vi "AO SCTR with Digital Out Engine.vi"(0 "Unique Notifier Name":string, 11 "AO PFI Lines":string[](array[string])) -> ()   [LabVIEW 2016]
uses:
  AO SCTR Type Defs/AO SCTR Notifier Type.ctl
  AO SCTR Type Defs/AO SCTR Actions.ctl
  <vilib>/DAQmx/write.llb/DAQmx Write (Analog DBL 1Chan 1Samp).vi
  <vilib>/Analysis/1siggen.llb/Ramp Pattern by Samples.vi
  <vilib>/DAQmx/write.llb/DAQmx Write (Analog 1D DBL 1Chan NSamp).vi
  <vilib>/DAQmx/create/channels.llb/DAQmx Create Channel (CO-Pulse Generation-Time).vi
  <vilib>/DAQmx/create/channels.llb/DAQmx Create Channel (AO-Voltage-Basic).vi
  <vilib>/DAQmx/miscellaneous.llb/DAQmx Fill In Error Info.vi
  <vilib>/DAQmx/configure/timing.llb/DAQmx Timing (Sample Clock).vi
  <resource>/objmgr/daqmx.rc
  <vilib>/Analysis/NI_AALBase.lvlib
panel:
  in  "Initial Delay":dbl format="%.6f"
  in  "Exposure Time (s)":dbl
  in  "Disable Input":bool
  out "Running":bool
  in  "Load":bool
  in  "Save":bool
  in  "Quit":bool
  in  "Waveform Settings":T1={"Actions"=enum."Stop at Offset", "Offset (V)"=-0.61, "Amplititude (V)"=0.524, "Samples Per Channel"=2280, "Start Delay (ms)"=20.0, "Running?"=FALSE} {"Amplititude (V)" format="%#_13g"; "Offset (V)" format="%#_13g"; "Start Delay (ms)" format="%#_13g"}
  out "Waveform Graph":dbl[](graph)
  out "Actual Sample Rate":dbl=10000.0 format="%0.2f"
  # "AO Line. Example: Dev1/ao1\nPFI (Trigger) Line. Example: /Dev1/PFI0\nCounter. Example: Dev1/ctr0"
  # "For debugging only."
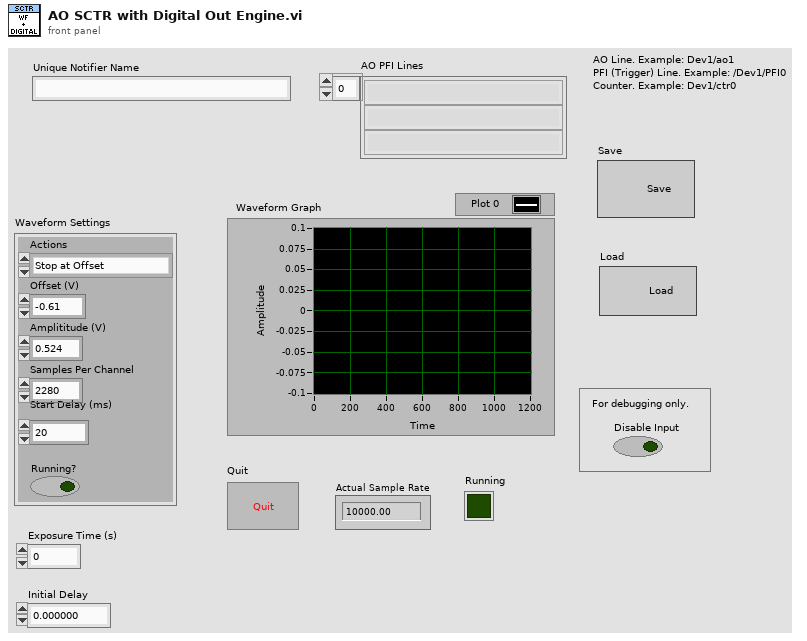
[diagram p1: front panel]
types:
  T1 = typedef "AO SCTR Notifier Type.ctl" = cluster{"Actions":T2, "Offset (V)":dbl, "Amplititude (V)":dbl, "Samples Per Channel":i32, "Start Delay (ms)":dbl, "Running?":bool}
  T2 = typedef "AO SCTR Actions.ctl" = enum16{"Stop at Offset", "Update and Run", "Quit"}
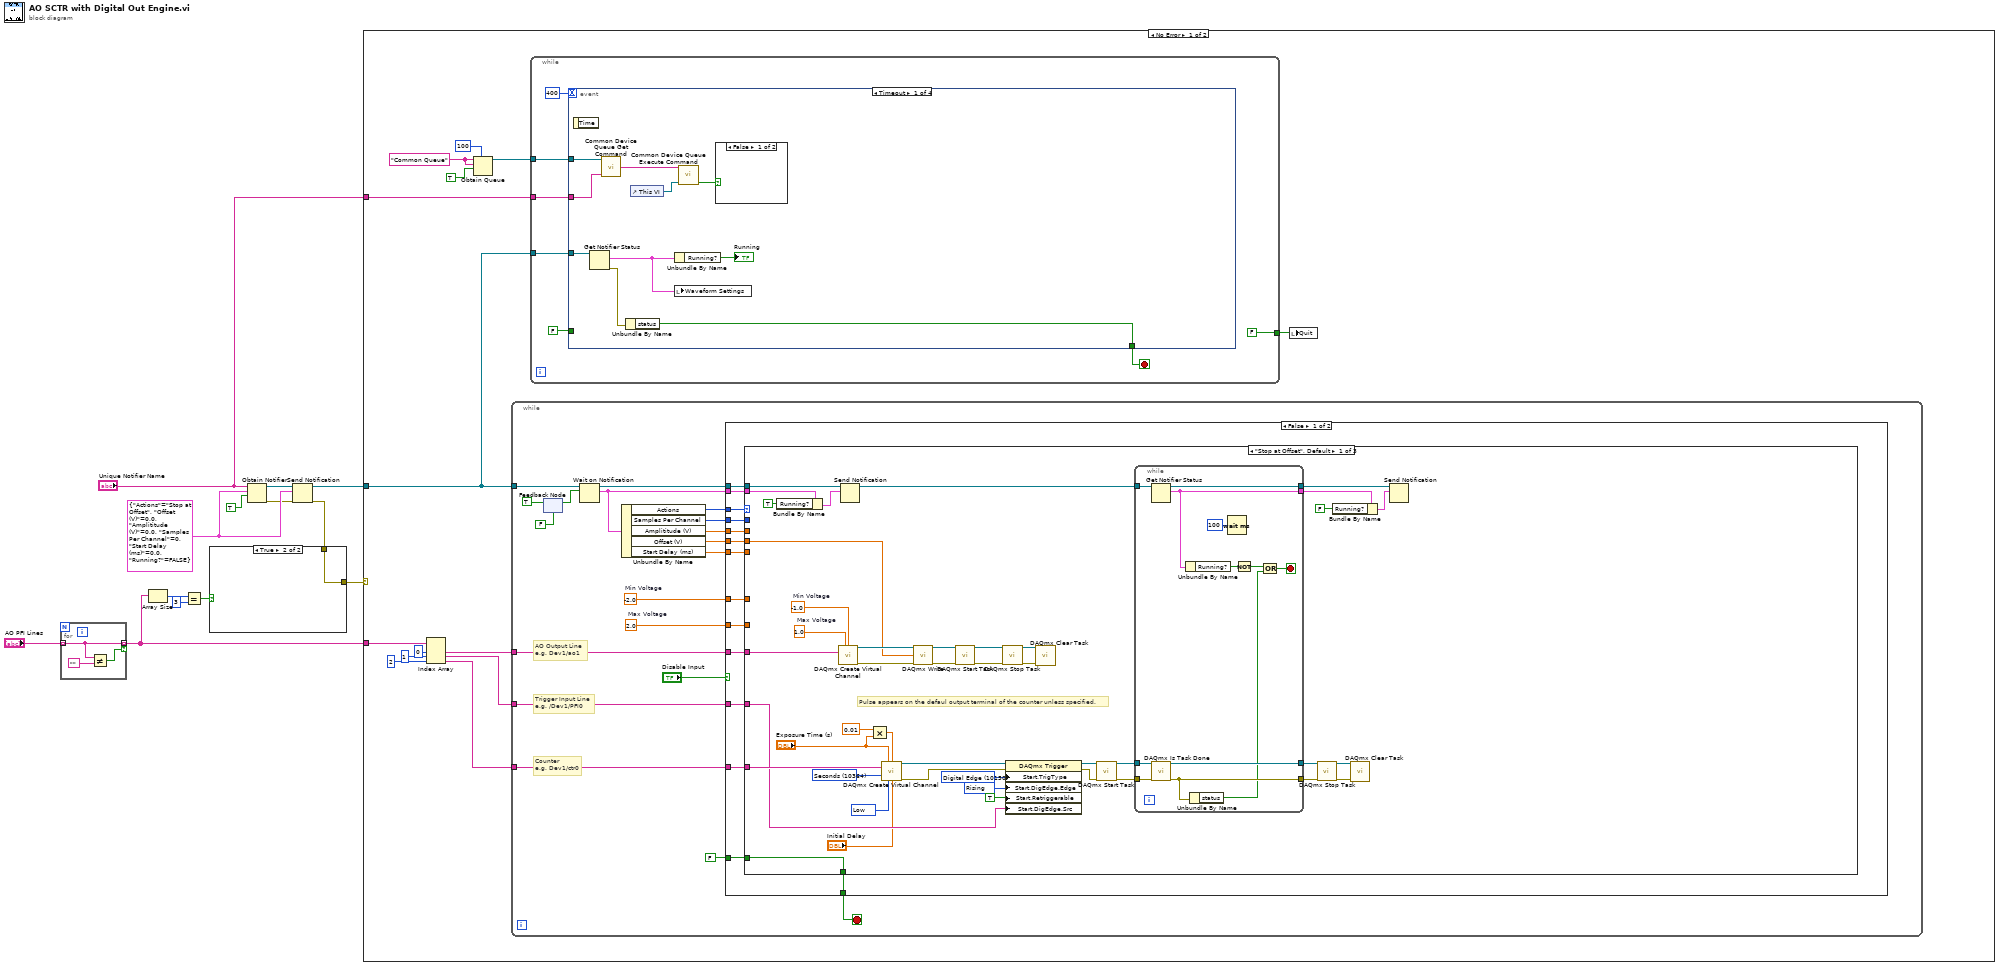
[diagram p0: block diagram]
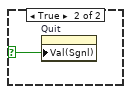
[diagram p2: hidden frame]
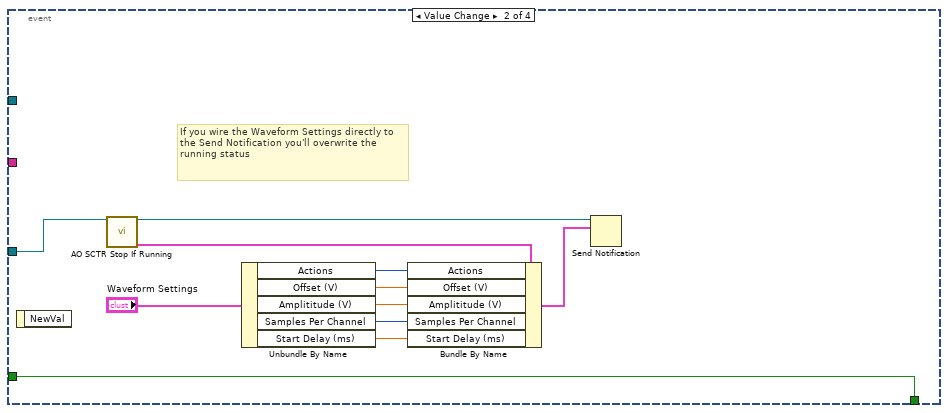
[diagram p3: hidden frame]
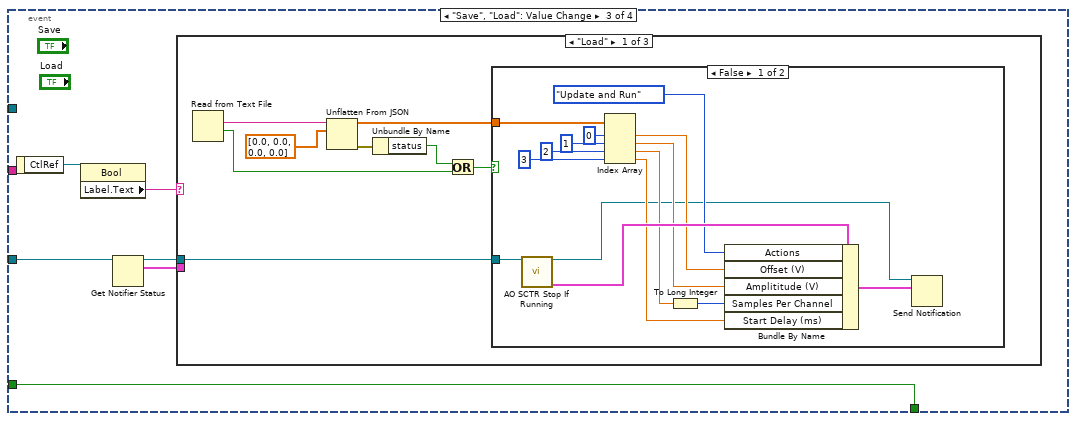
[diagram p4: hidden frame]
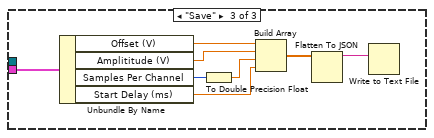
[diagram p7: hidden frame]
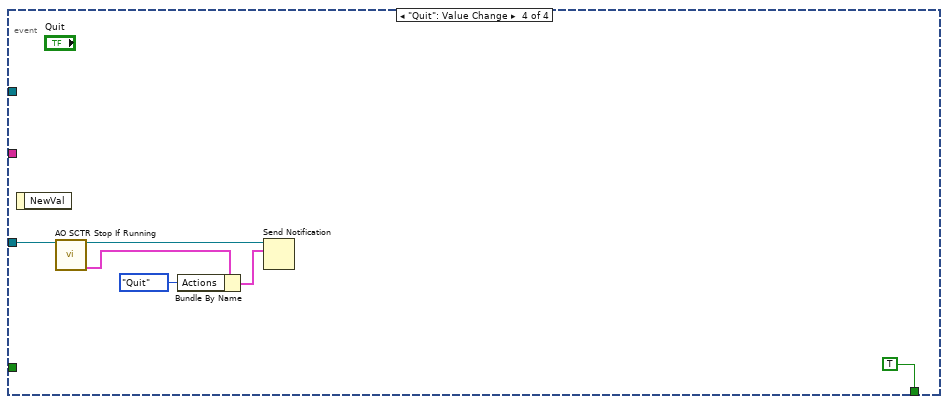
[diagram p8: hidden frame]
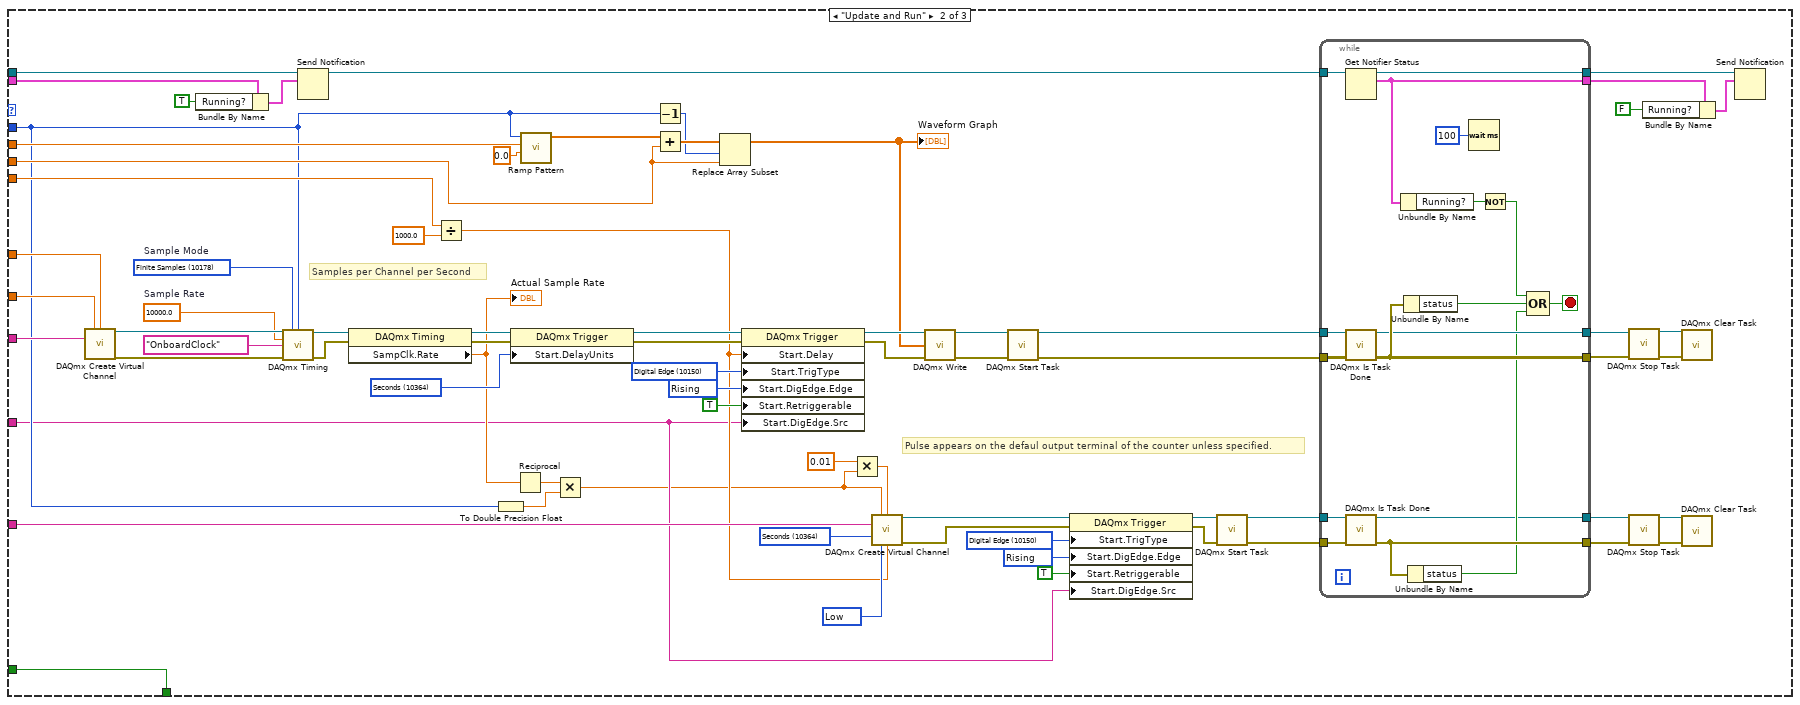
[diagram p9: hidden frame]
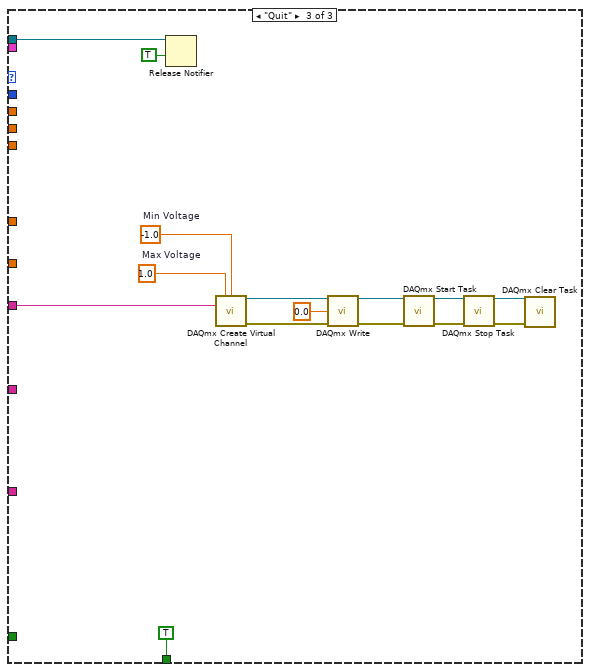
[diagram p10: hidden frame]
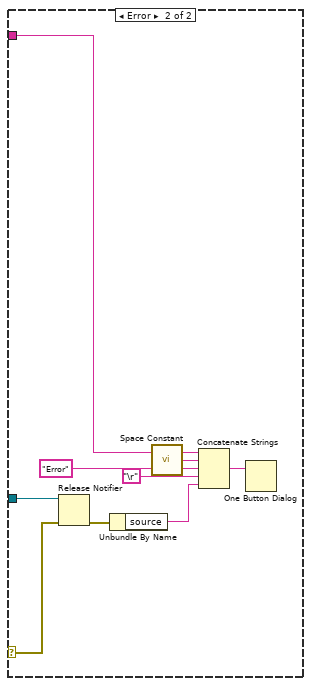
[diagram p12: hidden frame]
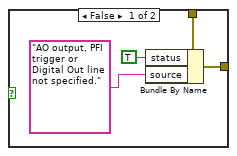
[diagram p13: hidden frame]
diagram:
  w8 = T1 {"Actions"=enum."Stop at Offset", "Offset (V)"=0.0, "Amplititude (V)"=0.0, "Samples Per Channel"=0, "Start Delay (ms)"=0.0, "Running?"=FALSE} ("Waveform Settings 2")
  n1 = for {
    tunnel: "AO PFI Lines" -> [w15] mode=indexing
    tunnel: [w15] -> w6 mode=indexing if=w14
    n2 = Not Equal?(x=w15, y="") -> (x != y?=w14:bool)
  }
  n3 = Array Size(array=w6) -> (size(s)=w5:i32)
  n4 = Equal?(x=w5, y=3) -> (x = y?=w3:bool)
  n5 = Obtain Notifier(name (unnamed)="Unique Notifier Name", notification data type=w8, create if not found? (T)=TRUE) -> (notifier out=w10:refnum<notifier>, error out=w7:errorcluster)  [unwired: 1 in, 1 out]
  n6 = Send Notification(notification=w8, notifier=w10, error in (no error)=w7) -> (notifier out=w9:refnum<notifier>, error out=w2:errorcluster)
  n7 = case shown="True" w3 {
    tunnel: w2 -> [w20 w21]
    tunnel: [w19 w21] -> w1
    frame False {
      n8 = Bundle By Name(cluster=w20, "status"=TRUE, "source"="AO output, PFI trigger or Digital Out line not specified.") -> (w19:errorcluster)
    }
    frame True {
    }
  }
  n9 = case shown="No Error" w1 {
    selector: w1 -> [_ w308]
    tunnel: "Unique Notifier Name" -> [w30 w306]
    tunnel: w9 -> [w25 w309]
    tunnel: w6 -> [w24 _]
    frame No Error {
      w35 = "Common Queue" ("Unique Notifier Name")
      n10 = Index Array(array=w24, index #1=0 ("index"), index #2=1 ("index"), index #3=2 ("index")) -> (element #1=w27:string, element #2=w26:string, element #3=w22:string)
      n11 = Obtain Queue(max queue size (-1, unlimited)=100, name (unnamed)=w35, element data type=w35, create if not found? (T)=TRUE) -> (queue out=w31:refnum<queue>)  [unwired: 1 in, 2 out]
      n12 = while {
        tunnel: w25 -> [w110]
        tunnel: w27 -> [w118]
        tunnel: w26 -> [w117]
        tunnel: w22 -> [w108]
        stop <- w119 stop-if-true
        w112 = 2.0  # Max Voltage
        w113 = -2.0  # Min Voltage
        # "Counter\ne.g. Dev1/ctr0"
        # "AO Output Line\ne.g. Dev1/ao1"
        # "Trigger Input Line\ne.g. /Dev1/PFI0"
        n13 = feedback-in #1(TRUE ("ignore previous (F)")) -> ()
        n14 = feedback #1(FALSE ("ignore previous (F)")) -> (w114:bool)
        n15 = Wait on Notification(notifier=w110, ignore previous (F)=w114) -> (notifier out=w121:refnum<notifier>, notification=w120:T1)  [unwired: 2 in, 2 out]
        n16 = Unbundle By Name(w120) -> ("Actions"=w122:T2, "Samples Per Channel"=w124:i32, "Amplititude (V)"=w126:dbl, "Offset (V)"=w123:dbl, "Start Delay (ms)"=w125:dbl)
        n17 = case shown="False" "Disable Input" {
          tunnel: w126 -> [w140 _]
          tunnel: w125 -> [w139 _]
          tunnel: w124 -> [w138 _]
          tunnel: w123 -> [w137 _]
          tunnel: w122 -> [w136 _]
          tunnel: w121 -> [w135 _]
          tunnel: w120 -> [w134 _]
          tunnel: [w133 w300] -> w119
          tunnel: w118 -> [w132 _]
          tunnel: w117 -> [w131 _]
          tunnel: w113 -> [w130 _]
          tunnel: w112 -> [w129 _]
          tunnel: FALSE -> [w128 w300]
          tunnel: w108 -> [w127 _]
          frame False {
            n18 = case shown="\"Stop at Offset\", Default" w136 {
              tunnel: w140 -> [_ w242 _]
              tunnel: w139 -> [_ w225 _]
              tunnel: w138 -> [_ w211 _]
              tunnel: w137 -> [w173 w241 _]
              tunnel: w135 -> [w151 w240 w297]
              tunnel: w134 -> [w149 w238 _]
              tunnel: [w172 w232 TRUE] -> w133
              tunnel: w132 -> [w171 w235 w285]
              tunnel: w131 -> [w158 w200 _]
              tunnel: w130 -> [_ w234 _]
              tunnel: w129 -> [_ w233 _]
              tunnel: w128 -> [w172 w232 _]
              tunnel: w127 -> [w159 w221 _]
              frame "Stop at Offset", Default {
                w167 = 10280 items=["Rising"=10280, "Falling"=10171] ("Start.DigEdge.Edge")
                w168 = 10150 items=["Analog Edge"=10099, "Analog Multi Edge"=16108, "Digital Edge"=10150, "Digital Pattern"=10398, "Analog Window"=10103, "Time"=15996, "None"=10230] ("Start.TrigType")
                w169 = 10214 items=["High"=10192, "Low"=10214] ("idle state")
                w170 = 10364 items=["Seconds"=10364] ("units")
                w175 = 1.0  # Max Voltage
                w174 = -1.0  # Min Voltage
                # "Pulse appears on the defaul output terminal of the counter unless specified."
                n19 = Bundle By Name(cluster=w149, "Running?"=TRUE ("Running")) -> (w152:T1)
                n20 = call-poly <vilib>:"DAQmx Create Virtual Channel.vi"("maximum value"=w175, "minimum value"=w174, "physical channels"=w171) -> ("task out"=w176:refnum<k21>, "error out"=w181:errorcluster)  [unwired: 11 in]
                n21 = Send Notification(notification=w152, notifier=w151) -> (notifier out=w150:refnum<notifier>)  [unwired: 1 in, 1 out]
                n22 = Multiply(x=0.01, y="Exposure Time (s)") -> (x*y=w143:dbl)
                n23 = call-poly <vilib>:"DAQmx Create Virtual Channel.vi"("high time"="Exposure Time (s)", "low time"=w143, "counter"=w159, "units"=w170, "idle state"=w169, "initial delay"="Initial Delay") -> ("task out"=w161:refnum<k21>, "error out"=w160:errorcluster)  [unwired: 8 in]
                n24 = call-poly <vilib>:"DAQmx Write.vi"("task/channels in"=w176, "data"=w173, "error in"=w181) -> ("task out"=w177:refnum<k21>, "error out"=w182:errorcluster)  [unwired: 10 in, 1 out]
                n25 = call <vilib>:"DAQmx Start Task.vi"("task/channels in"=w177, "error in"=w182) -> ("task out"=w179:refnum<k21>, "error out"=w183:errorcluster)  [unwired: 12 in]
                n26 = call <vilib>:"DAQmx Stop Task.vi"("task/channels in"=w179, "error in"=w183) -> ("task out"=w180:refnum<k21>, "error out"=w178:errorcluster)  [unwired: 12 in]
                n27 = property class="DAQmx Trigger"(reference=w161, error in=w160, "Start.TrigType"=w168, "Start.DigEdge.Edge"=w167, "Start.Retriggerable"=TRUE, "Start.DigEdge.Src"=w158) -> (reference out=w165:refnum<k21>, error out=w164:errorcluster)
                n28 = call <vilib>:"DAQmx Clear Task.vi"("task in"=w180, "error in"=w178) -> ()  [unwired: 13 in, 1 out]
                n29 = call <vilib>:"DAQmx Start Task.vi"("task/channels in"=w165, "error in"=w164) -> ("task out"=w155:refnum<k21>, "error out"=w154:errorcluster)  [unwired: 12 in]
                n30 = while {
                  tunnel: w150 -> [w195]
                  tunnel: w154 -> [w191]
                  tunnel: w155 -> [w192]
                  tunnel: [w190] -> w156
                  tunnel: [w189] -> w157
                  tunnel: [w185] -> w146
                  tunnel: [w184] -> w145
                  stop <- w186 stop-if-true
                  n31 = Get Notifier Status(notifier=w195) -> (notifier out=w185:refnum<notifier>, current notification=w184:T1)  [unwired: 1 in, 3 out]
                  n32 = call <vilib>:"DAQmx Is Task Done.vi"("task/channels in"=w192, "error in"=w191) -> ("task out"=w189:refnum<k21>, "error out"=w190:errorcluster)  [unwired: 11 in, 1 out]
                  n33 = Unbundle By Name(w184) -> ("Running?"=w194:bool)
                  n34 = Unbundle By Name(w190) -> ("status"=w187:bool)
                  n35 = Wait (ms)(milliseconds to wait=u32 100) -> ()  [unwired: 1 out]
                  n36 = Not(x=w194) -> (.not. x?=w188:bool)
                  n37 = Or(x=w188, y=w187) -> (x .or. y?=w186:bool)
                }
                n38 = call <vilib>:"DAQmx Stop Task.vi"("task/channels in"=w157, "error in"=w156) -> ("task out"=w162:refnum<k21>, "error out"=w163:errorcluster)  [unwired: 12 in]
                n39 = Bundle By Name(cluster=w145, "Running?"=FALSE ("Running")) -> (w147:T1)
                n40 = call <vilib>:"DAQmx Clear Task.vi"("task in"=w162, "error in"=w163) -> ()  [unwired: 13 in, 1 out]
                n41 = Send Notification(notification=w147, notifier=w146) -> ()  [unwired: 1 in, 2 out]
              }
              frame "Update and Run" {
                w216 = 10280 items=["Rising"=10280, "Falling"=10171] ("Start.DigEdge.Edge")
                w217 = 10150 items=["Analog Edge"=10099, "Analog Multi Edge"=16108, "Digital Edge"=10150, "Digital Pattern"=10398, "Analog Window"=10103, "Time"=15996, "None"=10230] ("Start.TrigType")
                w218 = 10214 items=["High"=10192, "Low"=10214] ("idle state")
                w219 = 10364 items=["Seconds"=10364] ("units")
                w227 = 10364 items=["Sample Clock Periods"=10286, "Seconds"=10364, "Ticks"=10304] ("Start.DelayUnits")
                w260 = 10000.0  # Sample Rate
                w252 = 10280 items=["Rising"=10280, "Falling"=10171] ("Start.DigEdge.Edge")
                w243 = 10150 items=["Analog Edge"=10099, "Digital Edge"=10150, "Digital Pattern"=10398, "Analog Window"=10103, "None"=10230] ("Start.TrigType")
                w266 = 10178 items=["Finite Samples"=10178, "Continuous Samples"=10123, "Hardware Timed Single Point"=12522]  # Sample Mode
                # "Pulse appears on the defaul output terminal of the counter unless specified."
                # "Samples per Channel per Second"
                n42 = call-poly <vilib>:"DAQmx Create Virtual Channel.vi"("maximum value"=w233, "minimum value"=w234, "physical channels"=w235) -> ("task out"=w264:refnum<k21>, "error out"=w265:errorcluster)  [unwired: 11 in]
                n43 = Bundle By Name(cluster=w238, "Running?"=TRUE ("Running")) -> (w236:T1)
                n44 = call-poly <vilib>:"DAQmx Timing.vi"("task/channels in"=w264, "sample mode"=w266, "samples per channel"=w211, "rate"=w260, "source"=tag "OnboardClock" ("Sample Clock Source"), "error in"=w265) -> ("task out"=w250:refnum<k21>, "error out"=w267:errorcluster)  [unwired: 8 in]
                n45 = Send Notification(notification=w236, notifier=w240) -> (notifier out=w239:refnum<notifier>)  [unwired: 1 in, 1 out]
                n46 = property class="DAQmx Timing"(reference=w250, error in=w267) -> (reference out=w226:refnum<k21>, error out=w222:errorcluster, "SampClk.Rate"=w213:dbl)
                "Actual Sample Rate" <- w213
                n47 = Divide(x=w225, y=1000.0) -> (x/y=w214:dbl)
                n48 = To Double Precision Float(number=w211) -> (double precision float=w210:dbl)
                n49 = property class="DAQmx Trigger"(reference=w226, error in=w222, "Start.DelayUnits"=w227) -> (reference out=w220:refnum<k21>, error out=w223:errorcluster)
                n50 = Reciprocal(x=w213) -> (1/x=w212:dbl)
                n51 = call-poly <vilib>:"Ramp Pattern.vi"("start"=0.0, "end"=w242, "samples"=w211) -> ("Ramp Pattern"=w247:dbl[])  [unwired: 7 in, 1 out]
                n52 = Multiply(x=w212, y=w210) -> (x*y=w199:dbl)
                n53 = Decrement(x=w211) -> (x-1=w245:i32)
                n54 = Add(x=w247, y=w241) -> (x+y=w246:dbl[])
                n55 = Replace Array Subset(array=w246, new element=w241, index=w245) -> (w244:dbl[])
                "Waveform Graph" <- w244
                n56 = property class="DAQmx Trigger"(reference=w220, error in=w223, "Start.Delay"=w214, "Start.TrigType"=w243, "Start.DigEdge.Edge"=w252, "Start.Retriggerable"=TRUE, "Start.DigEdge.Src"=w200) -> (reference out=w253:refnum<k21>, error out=w248:errorcluster)
                n57 = Multiply(x=0.01, y=w199) -> (x*y=w198:dbl)
                n58 = call-poly <vilib>:"DAQmx Create Virtual Channel.vi"("high time"=w199, "low time"=w198, "counter"=w221, "units"=w219, "idle state"=w218, "initial delay"=w214) -> ("task out"=w197:refnum<k21>, "error out"=w196:errorcluster)  [unwired: 8 in]
                n59 = call-poly <vilib>:"DAQmx Write.vi"("task/channels in"=w253, "data"=w244, "error in"=w248) -> ("task out"=w259:refnum<k21>, "error out"=w258:errorcluster)  [unwired: 10 in, 1 out]
                n60 = call <vilib>:"DAQmx Start Task.vi"("task/channels in"=w259, "error in"=w258) -> ("task out"=w263:refnum<k21>, "error out"=w262:errorcluster)  [unwired: 12 in]
                n61 = property class="DAQmx Trigger"(reference=w197, error in=w196, "Start.TrigType"=w217, "Start.DigEdge.Edge"=w216, "Start.Retriggerable"=TRUE, "Start.DigEdge.Src"=w200) -> (reference out=w208:refnum<k21>, error out=w207:errorcluster)
                n62 = call <vilib>:"DAQmx Start Task.vi"("task/channels in"=w208, "error in"=w207) -> ("task out"=w205:refnum<k21>, "error out"=w206:errorcluster)  [unwired: 12 in]
                n63 = while {
                  tunnel: w263 -> [w284]
                  tunnel: w262 -> [w283]
                  tunnel: [w282] -> w254
                  tunnel: [w281] -> w255
                  tunnel: w239 -> [w280]
                  tunnel: [w278] -> w231
                  tunnel: [w277] -> w228
                  tunnel: w206 -> [w274]
                  tunnel: w205 -> [w275]
                  tunnel: [w273] -> w201
                  tunnel: [w268] -> w202
                  stop <- w269 stop-if-true
                  n64 = Get Notifier Status(notifier=w280) -> (notifier out=w278:refnum<notifier>, current notification=w277:T1)  [unwired: 1 in, 3 out]
                  n65 = call <vilib>:"DAQmx Is Task Done.vi"("task/channels in"=w284, "error in"=w283) -> ("task out"=w281:refnum<k21>, "error out"=w282:errorcluster)  [unwired: 11 in, 1 out]
                  n66 = call <vilib>:"DAQmx Is Task Done.vi"("task/channels in"=w275, "error in"=w274) -> ("task out"=w268:refnum<k21>, "error out"=w273:errorcluster)  [unwired: 11 in, 1 out]
                  n67 = Unbundle By Name(w277) -> ("Running?"=w279:bool)
                  n68 = Unbundle By Name(w282) -> ("status"=w272:bool)
                  n69 = Unbundle By Name(w273) -> ("status"=w270:bool)
                  n70 = Wait (ms)(milliseconds to wait=u32 100) -> ()  [unwired: 1 out]
                  n71 = Not(x=w279) -> (.not. x?=w271:bool)
                  n72 = Compound Arithmetic op=OR(w271, w272, w270) -> (w269:bool)
                }
                n73 = call <vilib>:"DAQmx Stop Task.vi"("task/channels in"=w255, "error in"=w254) -> ("task out"=w257:refnum<k21>, "error out"=w256:errorcluster)  [unwired: 12 in]
                n74 = call <vilib>:"DAQmx Stop Task.vi"("task/channels in"=w202, "error in"=w201) -> ("task out"=w203:refnum<k21>, "error out"=w204:errorcluster)  [unwired: 12 in]
                n75 = Bundle By Name(cluster=w228, "Running?"=FALSE ("Running")) -> (w229:T1)
                n76 = call <vilib>:"DAQmx Clear Task.vi"("task in"=w257, "error in"=w256) -> ()  [unwired: 13 in, 1 out]
                n77 = call <vilib>:"DAQmx Clear Task.vi"("task in"=w203, "error in"=w204) -> ()  [unwired: 13 in, 1 out]
                n78 = Send Notification(notification=w229, notifier=w231) -> ()  [unwired: 1 in, 2 out]
              }
              frame "Quit" {
                w288 = 1.0  # Max Voltage
                w287 = -1.0  # Min Voltage
                n79 = Release Notifier(notifier=w297, force destroy? (F)=TRUE) -> ()  [unwired: 1 in, 3 out]
                n80 = call-poly <vilib>:"DAQmx Create Virtual Channel.vi"("maximum value"=w288, "minimum value"=w287, "physical channels"=w285) -> ("task out"=w289:refnum<k21>, "error out"=w294:errorcluster)  [unwired: 11 in]
                n81 = call-poly <vilib>:"DAQmx Write.vi"("task/channels in"=w289, "data"=0.0, "error in"=w294) -> ("task out"=w290:refnum<k21>, "error out"=w295:errorcluster)  [unwired: 10 in, 1 out]
                n82 = call <vilib>:"DAQmx Start Task.vi"("task/channels in"=w290, "error in"=w295) -> ("task out"=w292:refnum<k21>, "error out"=w296:errorcluster)  [unwired: 12 in]
                n83 = call <vilib>:"DAQmx Stop Task.vi"("task/channels in"=w292, "error in"=w296) -> ("task out"=w293:refnum<k21>, "error out"=w291:errorcluster)  [unwired: 12 in]
                n84 = call <vilib>:"DAQmx Clear Task.vi"("task in"=w293, "error in"=w291) -> ()  [unwired: 13 in, 1 out]
              }
            }
          }
          frame True {
          }
        }
      }
      n85 = while {
        tunnel: w25 -> [w42]
        tunnel: [FALSE] -> w32
        tunnel: w31 -> [w38]
        tunnel: w30 -> [w37]
        stop <- w40 stop-if-true
        n86 = event shown="[0] Timeout" {
          selector: _ -> [_ _ _ _]
          dyn-events: _ -> [_ _ _ _]
          timeout: 400 -> [_ _ _ _]
          tunnel: w42 -> [w52 w63 w68 w104]
          tunnel: [w50 w64 w65 TRUE ("status")] -> w40
          tunnel: w38 -> [w46 _ _ _]
          tunnel: w37 -> [w45 _ _ _]
          tunnel: FALSE ("status") -> [_ w64 w65 _]
          event Timeout {
            n87 = event-data() -> ()  [unwired: 1 in, 1 out]
            n88 = Get Notifier Status(notifier=w52) -> (current notification=w43:T1, error out=w51:errorcluster)  [unwired: 1 in, 3 out]
            n89 = call "Common Device Queue Get Command.vi"("Common Queue"=w46, "Notifier Name"=w45) -> ("Command"=w48:string)  [unwired: 12 in, 1 out]
            n90 = Unbundle By Name(w51) -> ("status"=w50:bool)
            n91 = control-ref of="This VI"() -> (w47:refnum<vi>)
            n92 = Unbundle By Name(w43) -> ("Running?"=→"Running":bool)
            n93 = local write "Waveform Settings"(w43) -> ()
            n94 = call "Common Device Queue Execute Command.vi"("Common Command"=w48, "VI Refnum"=w47) -> ("Quit?"=w49:bool)  [unwired: 12 in, 1 out]
            n95 = case shown="False" w49 {
              selector: w49 -> [_ w53]
              frame False {
              }
              frame True {
                n96 = property on="Quit" class="Bool (strict)"("Val(Sgnl)"=w53) -> ()  [unwired: 2 in, 2 out]
              }
            }
          }
          event Value Change {
            # "If you wire the Waveform Settings directly to the Send Notification you'll overwrite the running status"
            n97 = event-data() -> ()  [unwired: 1 in, 1 out]
            n98 = call "AO SCTR Stop If Running.vi"("AO SCTR Notifier"=w63) -> ("AO SCTR Notifier (Dup)"=w62:refnum<notifier>, "Latest Notification"=w61:T1)  [unwired: 13 in]
            n99 = Unbundle By Name("Waveform Settings") -> ("Actions"=w58:T2, "Offset (V)"=w57:dbl, "Amplititude (V)"=w56:dbl, "Samples Per Channel"=w55:i32, "Start Delay (ms)"=w54:dbl)
            n100 = Bundle By Name(cluster=w61, "Actions"=w58, "Offset (V)"=w57, "Amplititude (V)"=w56, "Samples Per Channel"=w55, "Start Delay (ms)"=w54) -> (w60:T1)
            n101 = Send Notification(notification=w60, notifier=w62) -> ()  [unwired: 1 in, 2 out]
          }
          event "Save", "Load": Value Change {
            n102 = event-data() -> ("CtlRef"=w70:refnum<vi>)  [unwired: 1 in]
            n103 = property class="Bool"(reference=w70) -> ("Label.Text"=w69:string)  [unwired: 1 in, 2 out]
            n104 = Get Notifier Status(notifier=w68) -> (notifier out=w66:refnum<notifier>, current notification=w67:T1)  [unwired: 1 in, 3 out]
            n105 = case shown="\"Load\"" w69 {
              tunnel: w67 -> [_ _ w101]
              tunnel: w66 -> [w72 _ _]
              frame "Load" {
                n106 = Read from Text File() -> (text=w78:string, cancelled=w74:bool)  [unwired: 4 in, 2 out]
                n107 = Unflatten From JSON(JSON string=w78, type and defaults=dbl[] [0.0, 0.0, 0.0, 0.0]) -> (value=w71:dbl[], error out=w76:errorcluster)  [unwired: 5 in]
                n108 = Unbundle By Name(w76) -> ("status"=w75:bool)
                n109 = Or(x=w75, y=w74) -> (x .or. y?=w73:bool)
                n110 = case shown="False" w73 {
                  tunnel: w72 -> [w93 _]
                  tunnel: w71 -> [w90 _]
                  frame False {
                    n111 = call "AO SCTR Stop If Running.vi"("AO SCTR Notifier"=w93) -> ("AO SCTR Notifier (Dup)"=w80:refnum<notifier>, "Latest Notification"=w92:T1)  [unwired: 13 in]
                    n112 = Index Array(array=w90, index #1=0 ("index"), index #2=1 ("index"), index #3=2 ("index"), index #4=3 ("index")) -> (element #1=w81:dbl, element #2=w82:dbl, element #3=w84:dbl, element #4=w85:dbl)
                    n113 = To Long Integer(number=w84) -> (32bit integer=w83:i32)
                    n114 = Bundle By Name(cluster=w92, "Actions"=AO_SCTR_Actions."Update and Run", "Offset (V)"=w81, "Amplititude (V)"=w82, "Samples Per Channel"=w83, "Start Delay (ms)"=w85) -> (w79:T1)
                    n115 = Send Notification(notification=w79, notifier=w80) -> ()  [unwired: 1 in, 2 out]
                  }
                  frame True {
                  }
                }
              }
              frame Default {
              }
              frame "Save" {
                n116 = Unbundle By Name(w101) -> ("Offset (V)"=w100:dbl, "Amplititude (V)"=w97:dbl, "Samples Per Channel"=w98:i32, "Start Delay (ms)"=w99:dbl)
                n117 = To Double Precision Float(number=w98) -> (double precision float=w96:dbl)
                n118 = Build Array(w100, w97, w96, w99) -> (w95:dbl[])
                n119 = Flatten To JSON(anything=w95) -> (JSON string=w94:string)  [unwired: 2 in, 1 out]
                n120 = Write to Text File(text=w94) -> ()  [unwired: 3 in, 3 out]
              }
            }
          }
          event "Quit": Value Change {
            n121 = event-data() -> ()  [unwired: 1 in, 1 out]
            n122 = call "AO SCTR Stop If Running.vi"("AO SCTR Notifier"=w104) -> ("AO SCTR Notifier (Dup)"=w103:refnum<notifier>, "Latest Notification"=w102:T1)  [unwired: 13 in]
            n123 = Bundle By Name(cluster=w102, "Actions"=AO_SCTR_Actions."Quit") -> (w106:T1)
            n124 = Send Notification(notification=w106, notifier=w103) -> ()  [unwired: 1 in, 2 out]
          }
        }
      }
      n125 = local write "Quit"(w32) -> ()
    }
    frame Error {
      n126 = Release Notifier(notifier=w309, error in (no error)=w308) -> (error out=w302:errorcluster)  [unwired: 1 in, 2 out]
      n127 = Unbundle By Name(w302) -> ("source"=w301:string)
      n128 = call <vilib>:"Space Constant.vi"() -> ("String"=w305:string)
      n129 = Concatenate Strings(w306, w305, "Error" ("string"), "\r", w301) -> (w307:string)
      n130 = One Button Dialog(message=w307) -> ()  [unwired: 1 in, 1 out]
    }
  }
